vi "Get Tree API.vi"(8 "error in (no error)":errorcluster, 11 "Brower View in":refnum<class "Brower View.lvclass">) -> (0 "error out":errorcluster, 2 "myTree.lvclass":refnum<class "MyTreeAPI.lvclass">, 3 "Brower View out":refnum<class "Brower View.lvclass">)   [LabVIEW 2015, in "Brower View.lvclass"]
uses:
  Brower View.lvclass
  MyTreeAPI/MyTreeAPI.lvclass
  Brower View.lvclass/Brower View.ctl
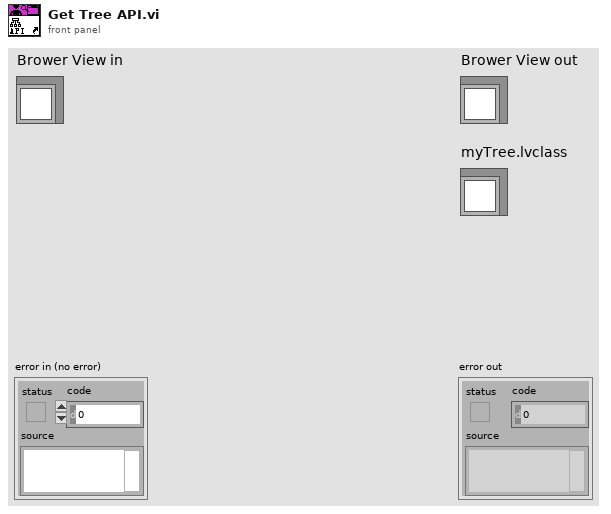
[diagram p1: front panel]
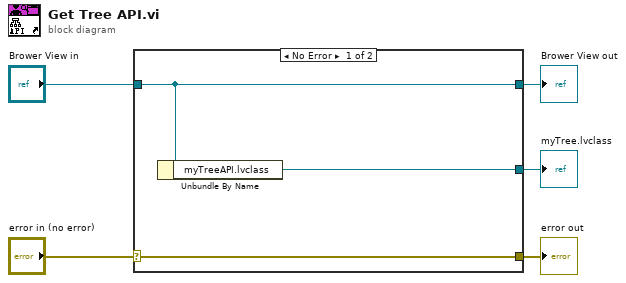
[diagram p0: block diagram]
diagram:
  n1 = case shown="No Error" "error in (no error)" {
    selector: "error in (no error)" -> [w8 w9]
    tunnel: [w8 w9] -> w4
    tunnel: [w7 w10] -> w2
    tunnel: "Brower View in" -> [w7 w10]
    tunnel: [w6 _] -> w1
    frame No Error {
      n2 = Unbundle By Name(w7) -> ("myTreeAPI.lvclass"=w6:refnum<class "MyTreeAPI.lvclass">)
    }
    frame Error {
    }
  }
  "error out" <- w4
  "Brower View out" <- w2
  "myTree.lvclass" <- w1
